vi "peakFinding whittakerSmooth.vi"(5 "diffMatrix":T1, 7 "lambda":i32=100, 10 "weight":dbl[](array[numeric]), 11 "data":dbl[](array[numeric])) -> (3 "background":dbl[](array[numeric]))   [LabVIEW 2018]
uses:
  <vilib>/Analysis/Matrix/Datatypes/RealMatrix.ctl
  <vilib>/Analysis/7linalg.llb/Real Transpose Matrix.vi
  <vilib>/Analysis/baseanly.llb/Real A x B.vi
  <vilib>/Analysis/Matrix/Numeric/Conversions/Array To Matrix - RA.vi
  <vilib>/Analysis/Matrix/Numeric/Multiply/Multiply - RM,R.vi
  <vilib>/Analysis/Matrix/Numeric/Add/Add - RM,RM.vi
  <vilib>/Analysis/7linalg.llb/Solve Linear Equations (multiple right hand).vi
  <vilib>/Analysis/Matrix/Numeric/Conversions/Matrix To Array - RM.vi
  <vilib>/Analysis/Matrix/NI_Matrix.lvlib
  <vilib>/Analysis/NI_AALPro.lvlib
  <vilib>/Analysis/NI_AALBase.lvlib
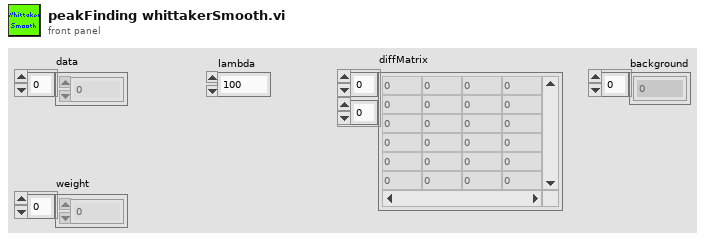
[diagram p1: front panel]
types:
  T1 = typedef "NI_Matrix.lvlib/RealMatrix.ctl" = dbl[][]
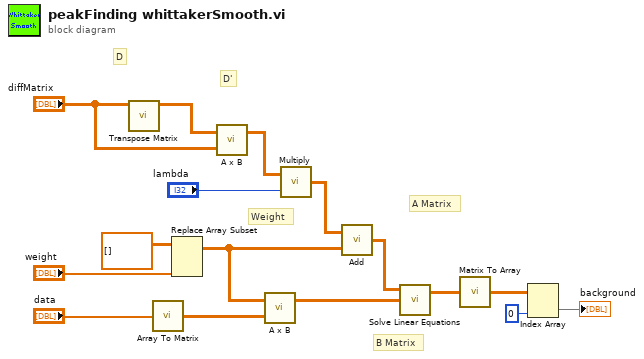
[diagram p0: block diagram]
diagram:
  # "B Matrix"
  # "A Matrix"
  # "Weight"
  # "D'"
  # "D"
  n1 = call-poly <vilib>:"Transpose Matrix.vi"("Input Matrix"="diffMatrix") -> ("Matrix Transpose"=w15:T1)  [unwired: 9 in, 1 out]
  n2 = call-poly <vilib>:"Array To Matrix.vi"("Real 1D Array"="data") -> ("Real Matrix (Column Vector)"=w10:T1)
  n3 = Replace Array Subset(array=T1 [] ("matrix"), new element="weight") -> (w11:T1)  [unwired: 2 in]
  n4 = call-poly <vilib>:"A x B.vi"("B"="diffMatrix", "A"=w15) -> ("A x B"=w14:T1)  [unwired: 1 out]
  n5 = call-poly <vilib>:"A x B.vi"("B"=w10, "A"=w11) -> ("A x B"=w8:T1)  [unwired: 1 out]
  n6 = call-poly <vilib>:"Multiply.vi"("Real Scalar c"="lambda", "Real Matrix A"=w14) -> ("A * c"=w12:T1)
  n7 = call-poly <vilib>:"Add.vi"("Real Matrix B"=w11, "Real Matrix A"=w12) -> ("A + B"=w9:T1)
  n8 = call-poly <vilib>:"Solve Linear Equations.vi"("Known Matrix"=w8, "Input Matrix"=w9) -> ("Solution Matrix"=w6:T1)  [unwired: 1 in, 1 out]
  n9 = call-poly <vilib>:"Matrix To Array.vi"("Real Matrix"=w6) -> ("Real 2D Array"=w5:dbl[][])
  n10 = Index Array(array=w5, index (col)=0 ("disabled index (col)")) -> (element=→"background":dbl[])  [unwired: 1 in]
